vi "AnalysisStats.vi"(9 "RFeArray":dbl[](array[numeric]), 10 "FeArray":dbl[](array[numeric]), 11 "TVEArray":dbl[](array[numeric])) -> (2 "StringArray":string[](array[string]), 3 "StatArray":dbl[](array[numeric]))   [LabVIEW 2014]
uses:
  <vilib>/Analysis/baseanly.llb/Mean (DBL).vi
  <vilib>/Analysis/NI_AALBase.lvlib
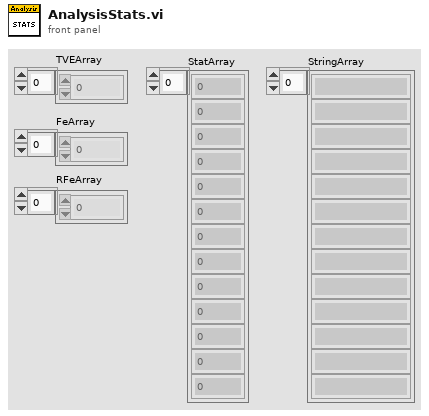
[diagram p1: front panel]
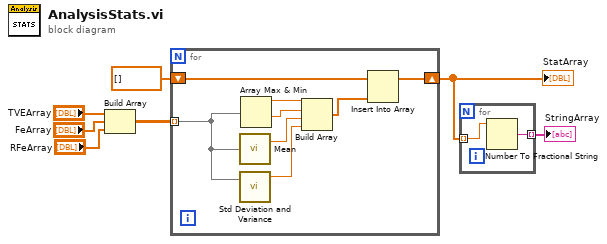
[diagram p0: block diagram]
diagram:
  n1 = Build Array("TVEArray", "FeArray", "RFeArray") -> (w7:dbl[][])
  n2 = for {
    shift-right: [w11] -> w3
    shift-left: dbl[] [] -> [w9]
    tunnel: w7 -> [w8] mode=indexing
    n3 = call-poly <vilib>:"Mean.vi"("X"=w8) -> ("mean"=w13:dbl)  [unwired: 1 out]
    n4 = call <vilib>:"Std Deviation and Variance.vi"("X"=w8) -> ("mean"=w12:dbl)  [unwired: 1 in, 2 out]
    n5 = Array Max & Min(array=w8) -> (max value=w15:dbl, min value=w14:dbl)  [unwired: 2 out]
    n6 = Build Array(w15, w14, w13, w12) -> (w10:dbl[])
    n7 = Insert Into Array(array=w9, new element=w10) -> (w11:dbl[])  [unwired: 1 in]
  }
  "StatArray" <- w3
  n8 = for {
    tunnel: w3 -> [w17] mode=indexing
    tunnel: [w16] -> w2 mode=indexing
    n9 = Number To Fractional String(number=w17) -> (F-format string=w16:string)  [unwired: 3 in]
  }
  "StringArray" <- w2
